vi "Process-error.vi"(8 "error in (no error)":errorcluster, 11 "Data in":T1) -> (0 "error out":errorcluster, 3 "Data out":T1)   [LabVIEW 2013, in "SLMControl.lvlib" / "SC-Main.lvclass"]
uses:
  SC-Main.lvclass
  Object-reference.ctl
  <vilib>/Utility/error.llb/DialogType.ctl
  Client/Sources/SC-Client.lvclass
  SM1000/SM1000.lvclass
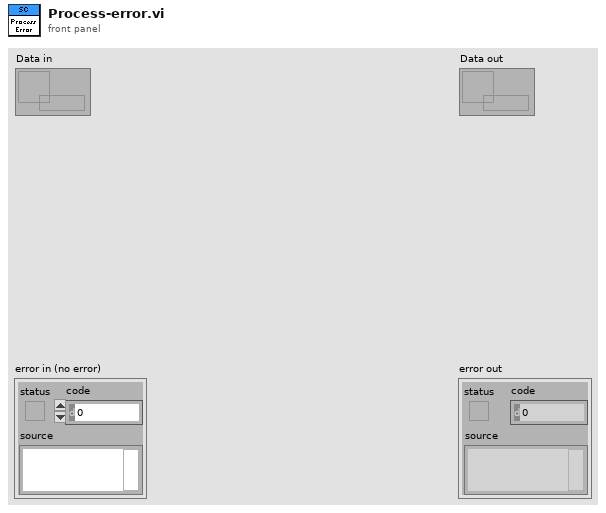
[diagram p1: front panel]
types:
  T1 = typedef "SLMControl.lvlib/SC-Main.lvclass/Object-reference.ctl" = refnum<data-value>
  T2 = typedef "DialogType.ctl" = u16
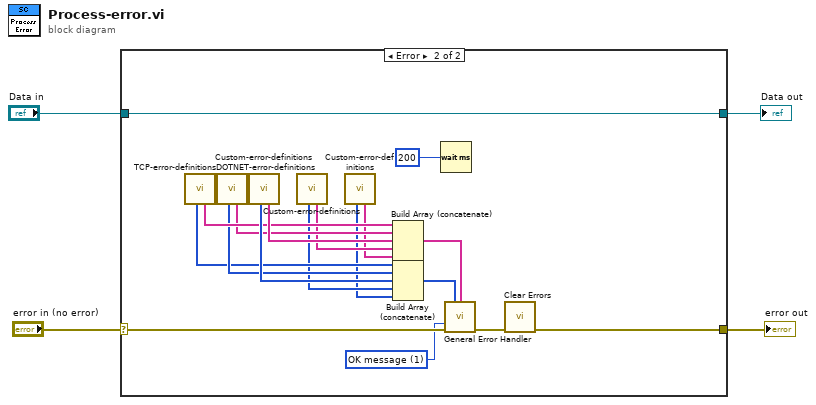
[diagram p0: block diagram]
diagram:
  n1 = case shown="Error" "error in (no error)" {
    selector: "error in (no error)" -> [w6 w24]
    tunnel: [w6 w21] -> w3
    tunnel: [w5 w23] -> w1
    tunnel: "Data in" -> [w5 w23]
    frame No Error {
    }
    frame Error {
      w20 = T2 1 items=["no dialog", "OK message", "continue or stop message", "OK message + warnings", "continue/stop + warnings"] ("type of dialog (OK msg:1)")
      n2 = call "TCP-error-definitions.vi"() -> ("Descriptions"=w14:string[], "Error codes"=w11:i32[])  [unwired: 10 in]
      n3 = call "DOTNET-error-definitions.vi"() -> ("Descriptions"=w13:string[], "Error codes"=w12:i32[])  [unwired: 10 in]
      n4 = call "Custom-error-definitions.vi"() -> ("Descriptions"=w17:string[], "Error codes"=w16:i32[])  [unwired: 10 in]
      n5 = call "Custom-error-definitions.vi"() -> ("Descriptions"=w10:string[], "Error codes"=w9:i32[])  [unwired: 9 in, 1 out]
      n6 = call "Custom-error-definitions.vi"() -> ("Descriptions"=w8:string[], "Error codes"=w7:i32[])  [unwired: 9 in, 1 out]
      n7 = Build Array (concatenate)(w14, w13, w17, w10, w8) -> (w19:string[])
      n8 = Build Array (concatenate)(w11, w12, w16, w9, w7) -> (w18:i32[])
      n9 = Wait (ms)(milliseconds to wait=u32 200) -> ()  [unwired: 1 out]
      n10 = call <vilib>:"General Error Handler.vi"("[user-defined codes]"=w18, "[user-defined descriptions]"=w19, "type of dialog (OK msg:1)"=w20, "error in (no error)"=w24) -> ("error out"=w22:errorcluster)  [unwired: 7 in, 4 out]
      n11 = call <vilib>:"Clear Errors.vi"("error in (no error)"=w22) -> ("error out"=w21:errorcluster)  [unwired: 6 in]
    }
  }
  "error out" <- w3
  "Data out" <- w1
